vi "Cleanup Write function.vi"(8 "error in (no error)":errorcluster, 9 "Project name":string, 11 "vi reference":refnum<vi>) -> (0 "error out":errorcluster, 3 "vi reference out":refnum<vi>)   [LabVIEW 2018]
doc: "Moves around controls and cleans up wires to make write accessors prettier."
uses:
  <vilib>/Utility/miscctls.llb/LVRectTypeDef.ctl
  <vilib>/Utility/miscctls.llb/LVPointTypeDef.ctl
  <vilib>/Utility/miscctls.llb/LVPositionTypeDef.ctl
  <vilib>/Utility/error.llb/Clear Errors.vi
  <userlib>/nLight Error Handling/Log any errors.vi
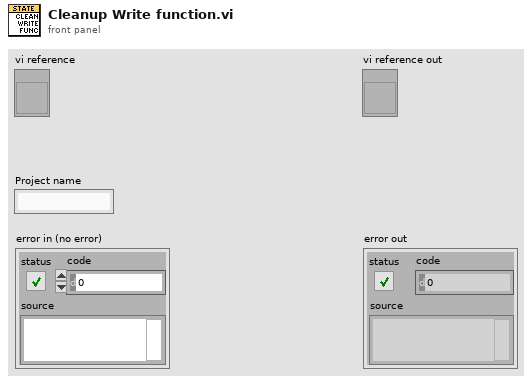
[diagram p1: front panel]
types:
  T1 = typedef "LVRectTypeDef.ctl" = cluster{"Left":i16, "Top":i16, "Right":i16, "Bottom":i16}
  T2 = typedef "LVPointTypeDef.ctl" = cluster{"Horizontal":i16, "Vertical":i16}
  T3 = cluster{"Label.Text":string, "Left":i32, "Top":i32}[]
  T4 = enum32{"Top Edges", "Vertical Centers", "Bottom Edges", "Left Edges", "Horizontal Centers", "Right Edges"}
  T5 = cluster{"Label.Text":string, "Left":i32, "Top":i32}
  T6 = typedef "LVPositionTypeDef.ctl" = cluster{"Left":i32, "Top":i32}
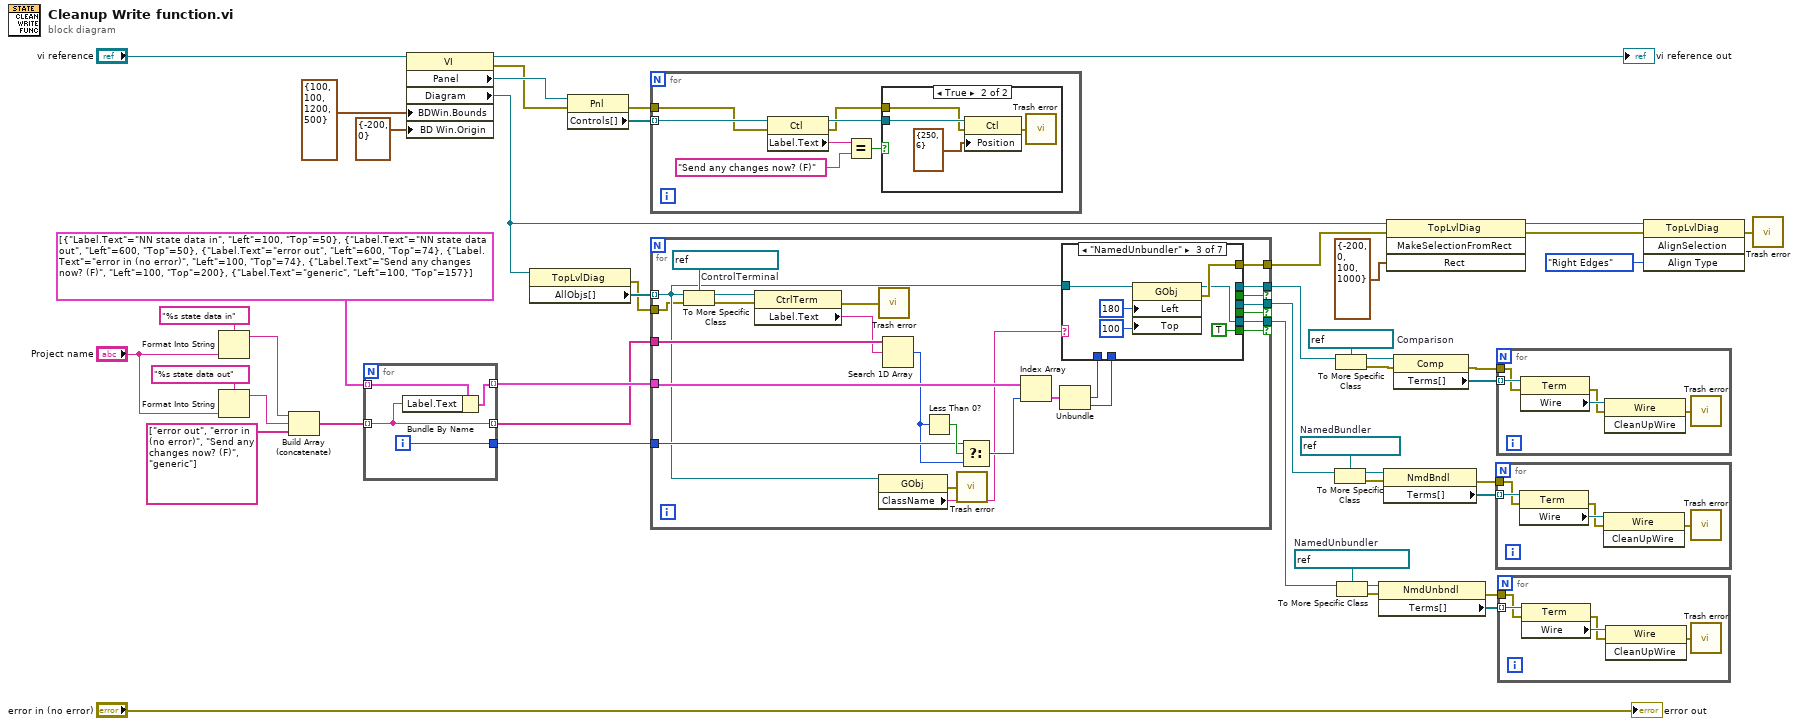
[diagram p0: block diagram]
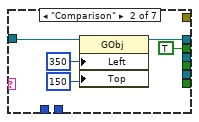
[diagram p4: hidden frame]
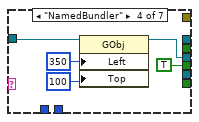
[diagram p5: hidden frame]
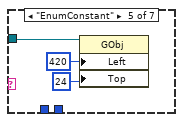
[diagram p6: hidden frame]
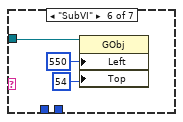
[diagram p7: hidden frame]
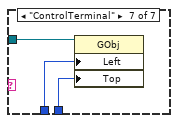
[diagram p8: hidden frame]
diagram:
  w29 = refnum<vi> refnum  # NamedBundler
  w30 = refnum<vi> refnum  # NamedUnbundler
  w42 = refnum<vi> refnum  # Comparison
  n1 = Format Into String(format string="%s state data in" ("Label.Text"), "Project name") -> (resulting string=w19:string)  [unwired: 2 in, 1 out]
  n2 = Format Into String(format string="%s state data out" ("Label.Text"), "Project name") -> (resulting string=w18:string)  [unwired: 2 in, 1 out]
  n3 = Build Array (concatenate)(w19, w18, string[] ["error out", "error in (no error)", "Send any changes now? (F)", "generic"] ("Label.Text")) -> (w17:string[])
  n4 = for {
    tunnel: T3 [{"Label.Text"="NN state data in", "Left"=100, "Top"=50}, {"Label.Text"="NN state data out", "Left"=600, "Top"=50}, {"Label.Text"="error out", "Left"=600, "Top"=74}, {"Label.Text"="error in (no error)", "Left"=100, "Top"=74}, {"Label.Text"="Send any changes now? (F)", "Left"=100, "Top"=200}, {"Label.Text"="generic", "Left"=100, "Top"=157}] ("Array") -> [w51] mode=indexing
    tunnel: [w48] -> w13 mode=indexing
    tunnel: [w49] -> w12
    tunnel: [w50] -> w14 mode=indexing
    tunnel: w17 -> [w48] mode=indexing
    i -> [w49]
    n5 = Bundle By Name(cluster=w51, "Label.Text"=w48) -> (w50:T5)
  }
  n6 = property class="VI"(reference="vi reference", "BDWin.Bounds"=T1 {"Left"=100, "Top"=100, "Right"=1200, "Bottom"=500} ("Block Diagram Window:Window Bounds"), "BD Win.Origin"=T2 {"Horizontal"=-200, "Vertical"=0} ("Block Diagram Window:Origin")) -> (reference out=→"vi reference out":refnum<vi>, error out=w11:errorcluster, "Panel"=w35:refnum<vi>, "Diagram"=w47:refnum<vi>)  [unwired: 1 in]
  n7 = property class="TopLvlDiag"(reference=w47) -> (error out=w9:errorcluster, "AllObjs[]"=w39:refnum<vi>[])  [unwired: 1 in, 1 out]
  n8 = property class="Pnl"(reference=w35, error in=w11) -> (error out=w10:errorcluster, "Controls[]"=w34:refnum<vi>[])  [unwired: 1 out]
  n9 = for {
    tunnel: w34 -> [w58] mode=indexing
    tunnel: w10 -> [w53]
    n10 = property class="Ctl"(reference=w58, error in=w53) -> (reference out=w55:refnum<vi>, error out=w52:errorcluster, "Label.Text"=w57:string)
    n11 = Equal?(x=w57, y="Send any changes now? (F)") -> (x = y?=w54:bool)
    n12 = case shown="True" w54 {
      tunnel: w55 -> [_ w62]
      tunnel: w52 -> [_ w60]
      frame False {
      }
      frame True {
        n13 = property class="Ctl"(reference=w62, error in=w60, "Position"=T6 {"Left"=250, "Top"=6}) -> (error out=w59:errorcluster)  [unwired: 1 out]
        n14 = call <userlib>:"Trash error.vi"("error in"=w59) -> ()  [unwired: 15 in]
      }
    }
  }
  n15 = for {
    tunnel: w39 -> [w75] mode=indexing
    tunnel: w14 -> [w84]
    tunnel: w13 -> [w86]
    tunnel: w12 -> [w79]
    tunnel: [w73] -> w43 if=w72
    tunnel: [w71] -> w36
    tunnel: [w70] -> w25 if=w69
    tunnel: [w68] -> w26 if=w67
    tunnel: w9 -> [w66]
    w76 = refnum<vi> refnum  # ControlTerminal
    n16 = To More Specific Class(target class=w76, reference=w75, error in=w66) -> (specific class reference=w87:refnum<vi>, error out=w65:errorcluster)
    n17 = property class="CtrlTerm"(reference=w87, error in=w65) -> (error out=w64:errorcluster, "Label.Text"=w85:string)  [unwired: 1 out]
    n18 = call <userlib>:"Trash error.vi"("error in"=w64) -> ()  [unwired: 15 in]
    n19 = property class="GObj"(reference=w75) -> (error out=w63:errorcluster, "ClassName"=w74:string)  [unwired: 1 in, 1 out]
    n20 = Search 1D Array(1D array=w86, element=w85) -> (index of element=w78:i32)  [unwired: 1 in]
    n21 = Less Than 0?(x=w78) -> (x < 0?=w80:bool)
    n22 = call <userlib>:"Trash error.vi"("error in"=w63) -> ()  [unwired: 15 in]
    n23 = Select(t=w79, s=w80, f=w78) -> (s? t:f=w77:i32)
    n24 = Index Array(array=w84, index=w77) -> (element=w83:T5)
    n25 = Unbundle(w83) -> ("Left"=w82:i32, "Top"=w81:i32)  [unwired: 1 out]
    n26 = case shown="\"NamedUnbundler\"" w74 {
      tunnel: w75 -> [_ w92 w98 w103 w106 w109 w112]
      tunnel: w82 -> [_ _ _ _ _ _ w111]
      tunnel: w81 -> [_ _ _ _ _ _ w110]
      tunnel: [_ w89 _ _ _ _ _] -> w73
      tunnel: [_ TRUE _ _ _ _ _] -> w72
      tunnel: [_ _ w95 _ _ _ _] -> w71
      tunnel: [_ _ w94 _ _ _ _] -> w68
      tunnel: [_ _ TRUE _ _ _ _] -> w67
      tunnel: [_ _ _ w100 _ _ _] -> w70
      tunnel: [_ _ _ TRUE _ _ _] -> w69
      frame Default {
      }
      frame "Comparison" {
        n27 = property class="GObj"(reference=w92, "Left"=350 ("Position:Left"), "Top"=150 ("Position:Top")) -> (reference out=w89:refnum<vi>)  [unwired: 1 in, 1 out]
      }
      frame "NamedUnbundler" {
        n28 = property class="GObj"(reference=w98, "Left"=180 ("Position:Left"), "Top"=100 ("Position:Top")) -> (reference out=w94:refnum<vi>, error out=w95:errorcluster)  [unwired: 1 in]
      }
      frame "NamedBundler" {
        n29 = property class="GObj"(reference=w103, "Left"=350 ("Position:Left"), "Top"=100 ("Position:Top")) -> (reference out=w100:refnum<vi>)  [unwired: 1 in, 1 out]
      }
      frame "EnumConstant" {
        n30 = property class="GObj"(reference=w106, "Left"=420 ("Position:Left"), "Top"=24 ("Position:Top")) -> ()  [unwired: 1 in, 2 out]
      }
      frame "SubVI" {
        n31 = property class="GObj"(reference=w109, "Left"=550 ("Position:Left"), "Top"=54 ("Position:Top")) -> ()  [unwired: 1 in, 2 out]
      }
      frame "ControlTerminal" {
        n32 = property class="GObj"(reference=w112, "Left"=w111, "Top"=w110) -> ()  [unwired: 1 in, 2 out]
      }
    }
  }
  n33 = To More Specific Class(target class=w29, reference=w25) -> (specific class reference=w28:refnum<vi>, error out=w2:errorcluster)  [unwired: 1 in]
  n34 = To More Specific Class(target class=w42, reference=w43) -> (specific class reference=w41:refnum<vi>, error out=w8:errorcluster)  [unwired: 1 in]
  n35 = To More Specific Class(target class=w30, reference=w26) -> (specific class reference=w31:refnum<vi>, error out=w1:errorcluster)  [unwired: 1 in]
  n36 = property class="NmdUnbndl"(reference=w31, error in=w1) -> (error out=w3:errorcluster, "Terms[]"=w32:refnum<vi>[])  [unwired: 1 out]
  n37 = property class="NmdBndl"(reference=w28, error in=w2) -> (error out=w4:errorcluster, "Terms[]"=w27:refnum<vi>[])  [unwired: 1 out]
  n38 = invoke class="TopLvlDiag" method="MakeSelectionFromRect"(reference=w47, error in=w36, "Rect"=T1 {"Left"=-200, "Top"=0, "Right"=100, "Bottom"=1000}) -> (reference out=w45:refnum<vi>, error out=w6:errorcluster)  [unwired: 1 in, 2 out]
  n39 = property class="Comp"(reference=w41, error in=w8) -> (error out=w7:errorcluster, "Terms[]"=w40:refnum<vi>[])  [unwired: 1 out]
  n40 = for {
    tunnel: w27 -> [w117] mode=indexing
    tunnel: w4 -> [w115]
    n41 = property class="Term"(reference=w117, error in=w115) -> (error out=w114:errorcluster, "Wire"=w116:refnum<vi>)  [unwired: 1 out]
    n42 = invoke class="Wire" method="CleanUpWire"(reference=w116, error in=w114) -> (error out=w113:errorcluster)  [unwired: 1 in, 2 out]
    n43 = call <userlib>:"Trash error.vi"("error in"=w113) -> ()  [unwired: 15 in]
  }
  n44 = for {
    tunnel: w40 -> [w122] mode=indexing
    tunnel: w7 -> [w120]
    n45 = property class="Term"(reference=w122, error in=w120) -> (error out=w119:errorcluster, "Wire"=w121:refnum<vi>)  [unwired: 1 out]
    n46 = invoke class="Wire" method="CleanUpWire"(reference=w121, error in=w119) -> (error out=w118:errorcluster)  [unwired: 1 in, 2 out]
    n47 = call <userlib>:"Trash error.vi"("error in"=w118) -> ()  [unwired: 15 in]
  }
  n48 = for {
    tunnel: w32 -> [w127] mode=indexing
    tunnel: w3 -> [w125]
    n49 = property class="Term"(reference=w127, error in=w125) -> (error out=w124:errorcluster, "Wire"=w126:refnum<vi>)  [unwired: 1 out]
    n50 = invoke class="Wire" method="CleanUpWire"(reference=w126, error in=w124) -> (error out=w123:errorcluster)  [unwired: 1 in, 2 out]
    n51 = call <userlib>:"Trash error.vi"("error in"=w123) -> ()  [unwired: 15 in]
  }
  n52 = invoke class="TopLvlDiag" method="AlignSelection"(reference=w45, error in=w6, "Align Type"=T4."Right Edges") -> (error out=w5:errorcluster)  [unwired: 1 in, 3 out]
  n53 = call <userlib>:"Trash error.vi"("error in"=w5) -> ()  [unwired: 15 in]
  "error out" <- "error in (no error)"
